vi "Consumer.vi"(8 "error in (no error)":errorcluster, 9 "Data":variant, 10 "Case ID":string, 11 "uService Template in":refnum<class "TCP Server.lvclass">) -> (0 "error out":errorcluster, 3 "uService Template out":refnum<class "TCP Server.lvclass">)   [LabVIEW 2026, in "TALOS.lvlib" / "TCP Server.lvlib" / "TCP Server.lvclass"]
uses:
  TCP Server.lvclass
  C:/LabVIEW Code/TALOS/talos/Father of all uServices/Father of all uServices/Father of all uServices.lvclass
  TCP Server Consumer Case Selector.ctl
  TCP Server.lvclass/TCP Server.ctl
  Ancestor/Ancestor/Ancestor.lvclass/Ancestor.ctl
  Father of all uServices/Father of all uServices Messages/Consumer Msg/Consumer Msg.lvclass/Consumer Msg.ctl
  Father of all uServices/Father of all uServices/Father of all uServices.lvclass/Father of all uServices.ctl
  Support VIs/Generate Error.vi
  Father of all uServices/Father of all uServices/Children Methods/Update GUI.vi
  FGV/Error Memory/Get Error Description.vi
  Support VIs/Get PC name.vi
  Ancestor/Ancestor/Read ID.vi
  Support VIs/Get Class Name.vi
  FGV/Error Memory/Error Memory Core.vi
  <vilib>/AdvancedString/Delimited String to 1D String Array.vi
  <vilib>/AdvancedString/Delimited String to 1D String Array (string).vi
  Support VIs/Circus Root Path.vi
  FGV/Error Memory/Error Crt Lvl checker.vi
  FGV/Error Memory/Error Memory Core.vi/40c8088d-b597-4017-91af-faa98e00292e.vi
  FGV/Error Memory/Error Memory Core.vi/d4a3ab98-063c-4e44-b43d-fbdcfe6c2be2.vi
  Father of all uServices/Father of all uServices/Father of all uServices.lvclass
  C:/LabVIEW Code/TALOS/builds/Actor Framework PPL/Actor Framework.lvlibp/1abvi3w/vi.lib/ActorFramework/Actor/Actor.lvclass
  Support VIs/Global Constants.vi
  Support VIs/Global Memory.vi
  <vilib>/Utility/LVClass/Get LV Class Name.vi
  Support VIs/Is in Packed Library.vi
  Support VIs/TALOS Root path.vi
  Support VIs/Read CSV worksheet.vi
  <vilib>/Utility/error.llb/General Error Handler.vi
  Support VIs/Error Log.vi
  builds/Actor Framework PPL/Actor Framework.lvlibp/1abvi3w/vi.lib/ActorFramework/Actor/Read Self Enqueuer.vi
  <userlib>/_OpenG.lib/lvdata/lvdata.llb/Get Strings from Enum__ogtk.vi
  builds/Actor Framework PPL/Actor Framework.lvlibp/1abvi3w/vi.lib/ActorFramework/Message Enqueuer/Enqueue.vi
  Father of all uServices/Father of all uServices/Children Methods/Get GUI Item Value - String.vi
  Father of all uServices/Father of all uServices/Multiline string updater.vi
  Ancestor/Ancestor/Ancestor.lvclass
  <vilib>/Comparison/Equal/Equal Functor/Equal Functor.lvclass
  Father of all uServices/Father of all uServices Messages/Consumer Msg/Consumer Msg.lvclass
  TALOS.lvlib
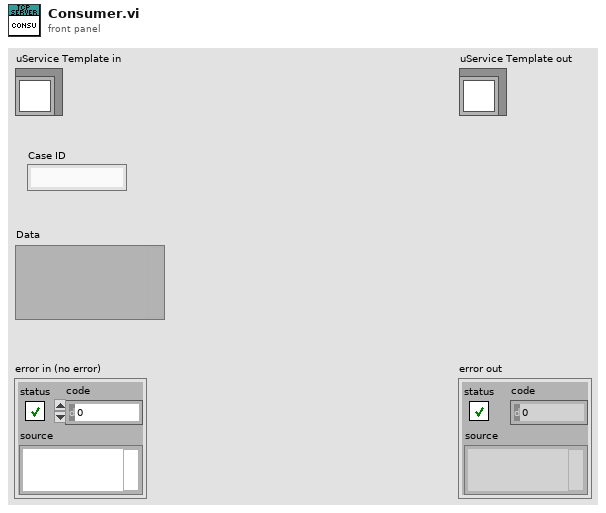
[diagram p1: front panel]
types:
  T1 = typedef "TALOS.lvlib/TCP Server.lvlib/TCP Server.lvclass/TCP Server Consumer Case Selector.ctl" = enum16{"Init", "Open Connection"}
  T2 = enum16{"Standard", "Buffered", "CRLF", "Immediate"}
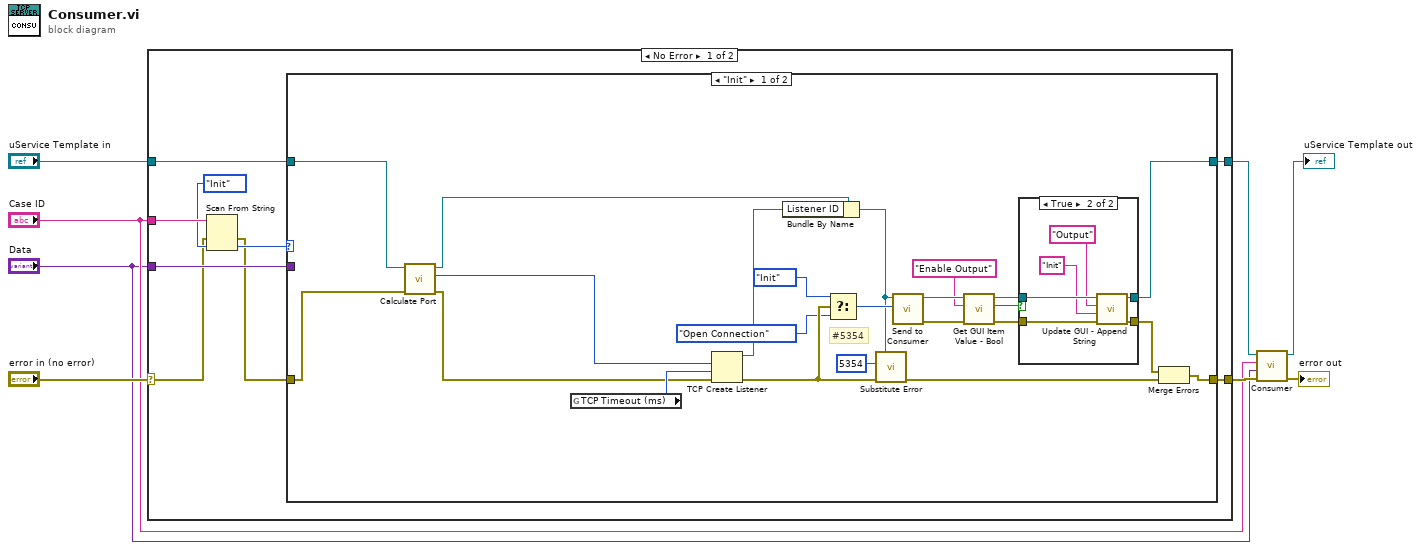
[diagram p0: block diagram]
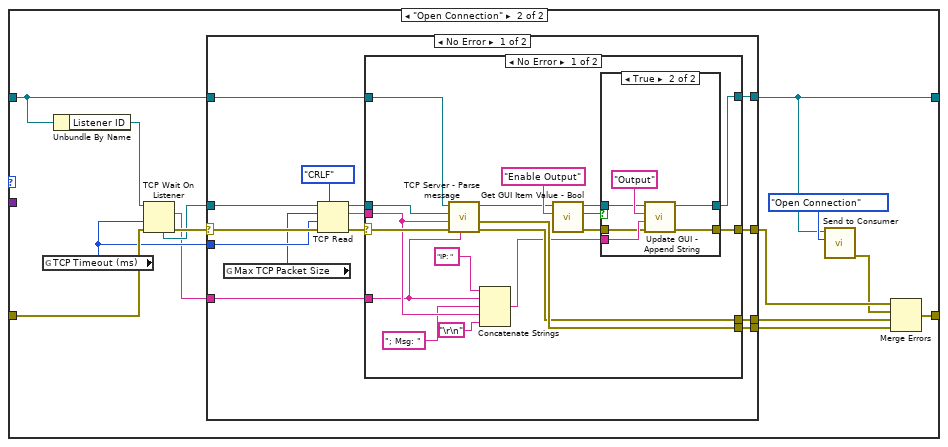
[diagram p3: hidden frame]
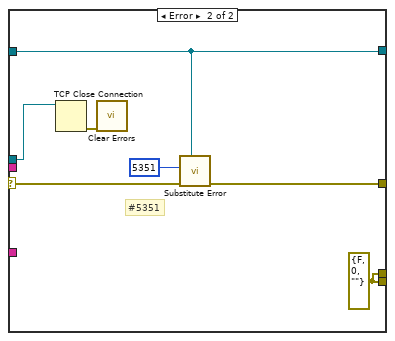
[diagram p5: hidden frame]
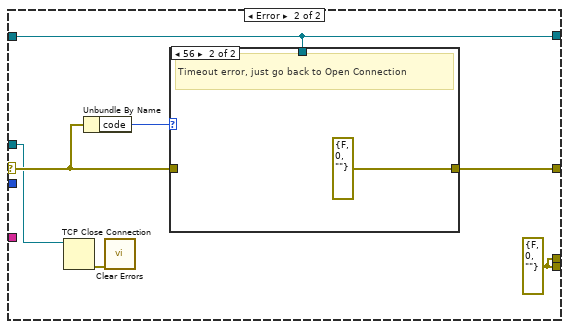
[diagram p6: hidden frame]
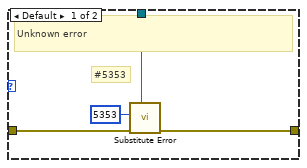
[diagram p7: hidden frame]
diagram:
  n1 = case shown="No Error" "error in (no error)" {
    selector: "error in (no error)" -> [w10 w122]
    tunnel: "uService Template in" -> [w16 w123]
    tunnel: [w14 w123] -> w4
    tunnel: [w15 w122] -> w3
    tunnel: "Case ID" -> [w13 _]
    tunnel: "Data" -> [w17 _]
    frame No Error {
      n2 = Scan From String(input string=w13, error in=w10, default 1=TCP_Server_Consumer_Case_Selector."Init") -> (error out=w9:errorcluster, output 1=w11:T1)  [unwired: 2 in, 2 out]
      n3 = case shown="\"Init\"" w11 {
        tunnel: w17 -> [_ _]
        tunnel: w9 -> [w22 w58]
        tunnel: w16 -> [w18 w53]
        tunnel: [w35 w55] -> w15
        tunnel: [w31 w54] -> w14
        frame "Init" {
          # "#5354"
          n4 = call-dynamic "Calculate Port.vi"("error in (no error)"=w22, "TCP Server in"=w18) -> ("error out"=w21:errorcluster, "Port"=w20:u16, "TCP Server out"=w19:refnum<class "TCP Server.lvclass">)  [unwired: 7 in]
          n5 = global read "Global Constants.vi" "TCP Timeout (ms)"() -> (w23:i32)
          n6 = TCP Create Listener(8:w21, 9:w23, 10:w20) -> (0:w40:errorcluster, 3:w36:refnum<k5>)  [unwired: 2 in, 1 out]
          n7 = Bundle By Name(cluster=w19, "Listener ID"=w36) -> (w33:refnum<class "TCP Server.lvclass">)
          n8 = Select(t=TCP_Server_Consumer_Case_Selector."Init", s=w40, f=TCP_Server_Consumer_Case_Selector."Open Connection") -> (s? t:f=w37:T1)
          n9 = call "Substitute Error.vi"("LabVIEW Object"=w33, "error in (no error)"=w40, "Error Code"=5354) -> ("error out"=w34:errorcluster)  [unwired: 8 in]
          n10 = call "Send to Consumer.vi"("Case ID"=w37, "uService Template in"=w33) -> ("error out"=w28:errorcluster, "uService Template out"=w29:refnum<class "TCP Server.lvclass">)  [unwired: 8 in]
          n11 = call "Get GUI Item Value - Bool.vi"("error in (no error)"=w28, "FP Item Name"="Enable Output" ("Parameter Name"), "uService Template in"=w29) -> ("error out"=w27:errorcluster, "Value"=w26:bool, "uService Template out"=w25:refnum<class "TCP Server.lvclass">)  [unwired: 6 in]
          n12 = case shown="True" w26 {
            tunnel: w25 -> [w42 w48]
            tunnel: [w42 w47] -> w31
            tunnel: [w41 w46] -> w30
            tunnel: w27 -> [w41 w43]
            frame False {
            }
            frame True {
              n13 = call "Update GUI - Append String.vi"("error in (no error)"=w43, "String"="Init", "GUI Item Name"="Output", "Father of all uServices in"=w48) -> ("error out"=w46:errorcluster, "Father of all uServices out"=w47:refnum<class "TCP Server.lvclass">)  [unwired: 6 in]
            }
          }
          n14 = Merge Errors(w30, w34) -> (w35:errorcluster)
        }
        frame "Open Connection" {
          n15 = global read "Global Constants.vi" "TCP Timeout (ms)"() -> (w52:i32)
          n16 = Unbundle By Name(w53) -> ("Listener ID"=w59:refnum<k5>)
          n17 = TCP Wait On Listener(8:w58, 9:w52, 11:w59) -> (0:w62:errorcluster, 2:w51:string, 4:w61:refnum<k5>)  [unwired: 1 in, 2 out]
          n18 = case shown="No Error" w62 {
            selector: w62 -> [w76 w114]
            tunnel: w61 -> [w75 w111]
            tunnel: [w70 w115] -> w57
            tunnel: w53 -> [w69 w113]
            tunnel: [w68 w113] -> w54
            tunnel: w52 -> [w67 _]
            tunnel: w51 -> [w65 _]
            tunnel: [w64 w112] -> w50
            tunnel: [w63 w112] -> w49
            frame No Error {
              n19 = global read "Global Constants.vi" "Max TCP Packet Size"() -> (w66:i32)
              n20 = TCP Read(connection ID=w75, bytes to read=w66, error in (no error)=w76, 7:T2."CRLF" ("mode (standard)"), 9:w67) -> (connection ID out=w72:refnum<k5>, data out=w71:string, error out=w73:errorcluster)
              n21 = case shown="No Error" w73 {
                selector: w73 -> [w94 w108]
                tunnel: w72 -> [w92 w103]
                tunnel: w71 -> [w90 _]
                tunnel: [w89 w107] -> w70
                tunnel: w69 -> [w93 w106]
                tunnel: [w88 w106] -> w68
                tunnel: w65 -> [w79 _]
                tunnel: [w80 w105] -> w64
                tunnel: [w78 w105] -> w63
                frame No Error {
                  n22 = call "TCP Server - Parse message.vi"("Sender IP"=w79, "error in (no error)"=w94, "Message"=w90, "TCP Client ID"=w92, "TCP Server in"=w93) -> ("error out"=w78:errorcluster, "External error out"=w80:errorcluster, "TCP Server out"=w82:refnum<class "TCP Server.lvclass">)  [unwired: 4 in]
                  n23 = Concatenate Strings("IP: " ("string"), w79, "; Msg: " ("string"), w90, "\r\n") -> (w77:string)
                  n24 = call "Get GUI Item Value - Bool.vi"("FP Item Name"="Enable Output" ("Parameter Name"), "uService Template in"=w82) -> ("error out"=w84:errorcluster, "Value"=w83:bool, "uService Template out"=w81:refnum<class "TCP Server.lvclass">)  [unwired: 7 in]
                  n25 = case shown="True" w83 {
                    tunnel: [w95 w102] -> w89
                    tunnel: [w96 w99] -> w88
                    tunnel: w81 -> [w96 w100]
                    tunnel: w77 -> [_ w98]
                    tunnel: w84 -> [w95 w97]
                    frame False {
                    }
                    frame True {
                      n26 = call "Update GUI - Append String.vi"("error in (no error)"=w97, "String"=w98, "GUI Item Name"="Output", "Father of all uServices in"=w100) -> ("error out"=w102:errorcluster, "Father of all uServices out"=w99:refnum<class "TCP Server.lvclass">)  [unwired: 6 in]
                    }
                  }
                }
                frame Error {
                  w105 = errorcluster {"status"=FALSE, "code"=0, "source"=""} ("External error out")
                  # "#5351"
                  n27 = TCP Close Connection(connection ID=w103) -> (error out=w104:errorcluster)  [unwired: 2 in, 1 out]
                  n28 = call <vilib>:"Clear Errors.vi"("error in (no error)"=w104) -> ()  [unwired: 5 in, 2 out]
                  n29 = call "Substitute Error.vi"("LabVIEW Object"=w106, "error in (no error)"=w108, "Error Code"=5351) -> ("error out"=w107:errorcluster)  [unwired: 8 in]
                }
              }
            }
            frame Error {
              w112 = errorcluster {"status"=FALSE, "code"=0, "source"=""} ("External error out")
              n30 = TCP Close Connection(connection ID=w111) -> (error out=w110:errorcluster)  [unwired: 2 in, 1 out]
              n31 = Unbundle By Name(w114) -> ("code"=w116:i32)
              n32 = call <vilib>:"Clear Errors.vi"("error in (no error)"=w110) -> ()  [unwired: 5 in, 2 out]
              n33 = case shown="56" w116 {
                tunnel: [w119 errorcluster {"status"=FALSE, "code"=0, "source"=""} ("error IO")] -> w115
                tunnel: w114 -> [w120 _]
                tunnel: w113 -> [w118 _]
                frame Default {
                  # "#5353"
                  # "Unknown error"
                  n34 = call "Substitute Error.vi"("LabVIEW Object"=w118, "error in (no error)"=w120, "Error Code"=5353) -> ("error out"=w119:errorcluster)  [unwired: 8 in]
                }
                frame 56 {
                  # "Timeout error, just go back to Open Connection"
                }
              }
            }
          }
          n35 = call "Send to Consumer.vi"("Case ID"=TCP_Server_Consumer_Case_Selector."Open Connection", "uService Template in"=w54) -> ("error out"=w56:errorcluster)  [unwired: 8 in, 1 out]
          n36 = Merge Errors(w57, w56, w49, w50) -> (w55:errorcluster)
        }
      }
    }
    frame Error {
    }
  }
  n37 = call-parent "Consumer.vi"("error in (no error)"=w3, "Data"="Data", "Case ID"="Case ID", "uService Template in"=w4) -> ("error out"=→"error out":errorcluster, "uService Template out"=→"uService Template out":refnum<class "TCP Server.lvclass">)  [unwired: 6 in]
